vi "Read secondsArc.vi"(8 "error in (no error)":errorcluster, 11 "Declination in":refnum<class "Declination.lvclass">) -> (0 "error out":errorcluster, 2 "secondsArc":dbl[unit] min=0.0 max=0.0002908882086657216, 3 "Declination out":refnum<class "Declination.lvclass">)   [LabVIEW 2022 SP3, in "TCSDataDefinitions.lvlib" / "TCSCommand.lvlib" / "TargetConfiguration.lvlib" / "Target.lvlib" / "FixedTarget.lvlib" / "Declination.lvclass"]
uses:
  Declination.lvclass
  Declination.lvclass/Declination.ctl
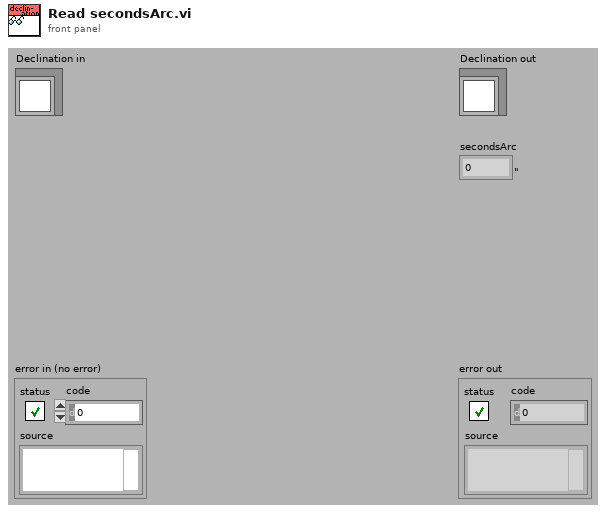
[diagram p1: front panel]
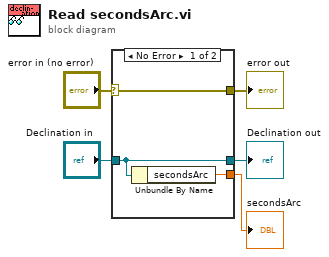
[diagram p0: block diagram]
diagram:
  n1 = case shown="No Error" "error in (no error)" {
    selector: "error in (no error)" -> [w8 w9]
    tunnel: [w8 w9] -> w4
    tunnel: [w7 w10] -> w2
    tunnel: "Declination in" -> [w7 w10]
    tunnel: [w6 _] -> w1
    frame No Error {
      n2 = Unbundle By Name(w7) -> ("secondsArc"=w6:dbl[unit])
    }
    frame Error {
    }
  }
  "error out" <- w4
  "Declination out" <- w2
  "secondsArc" <- w1
